vi "updateChannelControls.vi"(10 "Cluster":T1={"rigChannels"=[], "rigUnits"=[], "logging"=FALSE, "chartRef"=refnum, "dataTableRef"=refnum, "channelCount"=0, "trendIndex"=0, "channels"={"massflow"=0, "PR"=0, "recircTemp"=0}, "History"={"speedlines"=[], "liveTail"={"mDot"=[], "pRatio"=[]}, "current"={"mDot"=0.0, "pRatio"=0.0}, "insertPoint"=0, "tempHistory"=[]}, "filter"=FALSE, "filterLength"=0, "tableUpdate"=0, "limitValues"=[[0.0, 45000.0], [0.0, 100.0], [0.0, 100.0], [10.0, 100.0], [0.0, 100.0], [10.0, 35.0], [0.0, 100.0], [0.0, 100.0], [99000.0, 300000.0], [-5000.0, 5000.0], [99000.0, 300000.0], [-0.01, 0.3], [-0.01, 4.5], [-0.1, 100.0], [1.0, 8.0], [1.0, 5.0], [0.0, 100.0], [0.0, 100.0], [0.0, 100.0], [-100.0, 45000.0], [-0.1, 1.0], [0.8, 2.0], [90000.0, 110000.0], [15.0, 35.0], [0.0, 0.0], [0.0, 0.0], [0.0, 0.0], [0.0, 0.0]]}, 11 "channels":refnum<vi>) -> ()   [LabVIEW 2018]
uses:
  custom sub vis/speedlineData.ctl
panel:
  out "error out":errorcluster
  in  "Ring":i32(ring)
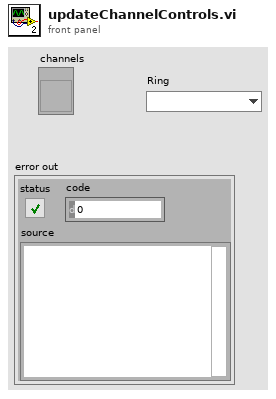
[diagram p1: front panel]
types:
  T1 = typedef "speedlineData.ctl" = cluster{"rigChannels":string[], "rigUnits":string[], "logging":bool, "chartRef":refnum<vi>, "dataTableRef":refnum<vi>, "channelCount":i32, "trendIndex":i32, "channels":cluster{"massflow":i32, "PR":i32, "recircTemp":i32}, "History":cluster{"speedlines":cluster{"mDot":dbl[], "pRatio":dbl[]}[], "liveTail":cluster{"mDot":dbl[], "pRatio":dbl[]}, "current":cluster{"mDot":dbl, "pRatio":dbl}, "insertPoint":i32, "tempHistory":dbl[][]}, "filter":bool, "filterLength":i32, "tableUpdate":i16, "limitValues":dbl[][]}
  T2 = cluster{"massflow":i32, "PR":i32, "recircTemp":i32}
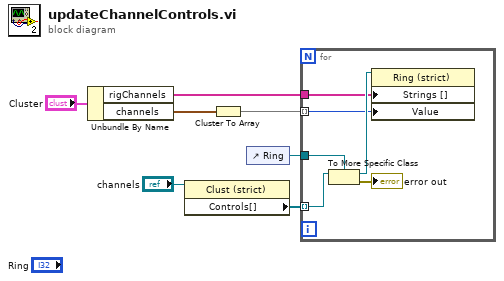
[diagram p0: block diagram]
diagram:
  n1 = Unbundle By Name("Cluster") -> ("rigChannels"=w4:string[], "channels"=w3:T2)
  n2 = property class="Clust (strict)"(reference="channels") -> ("Controls[]"=w6:refnum<vi>[])  [unwired: 1 in, 2 out]
  n3 = Cluster To Array(cluster=w3) -> (array=w2:i32[])
  n4 = control-ref of="Ring"() -> (w5:refnum<vi>)
  n5 = for {
    tunnel: w6 -> [w10] mode=indexing
    tunnel: w5 -> [w12]
    tunnel: w4 -> [w11]
    tunnel: w2 -> [w8] mode=indexing
    n6 = To More Specific Class(target class=w12, reference=w10) -> (specific class reference=w13:refnum<vi>, error out=→"error out":errorcluster)  [unwired: 1 in]
    n7 = property class="Ring (strict)"(reference=w13, "Strings []"=w11, "Value"=w8) -> ()  [unwired: 1 in, 2 out]
  }
